vi "TAT_Com_PLC.vi"() -> ()   [LabVIEW 2017]
uses:
  NIVISION/Kapse And Sons/CKD POKAYOKE TRACIBILITY/Controls/PLC_Comm_State.ctl
  <vilib>/NI/Modbus Library/API/Master/Modbus Master.lvclass
  Global/PLC_to_Auto.vi
  <vilib>/NI/Modbus Library/API/Wrapper/Create TCP Master.vi
  <vilib>/NI/Modbus Library/API/Wrapper/API Main.lvlib
panel:
  out "s? t:f":T1
  out "Feeder Door Open":cluster{"Feeder Door Open":bool, "Address":u16}
  out "PLC IP Address":string
  out "error out 2":errorcluster
  out "error IO":errorcluster
  in  "stop 2":bool
  out "PLC STATUS station 2":bool
  out "error IO 2":errorcluster
  out "Latch Error Case":errorcluster
  out "I/O SCREEN":bool[](array[boolean])
  out "error out":errorcluster
  in  "PLC STATUS station 1":bool
  in  "error in":errorcluster
  in  "stop":bool
  # "STATION 1"
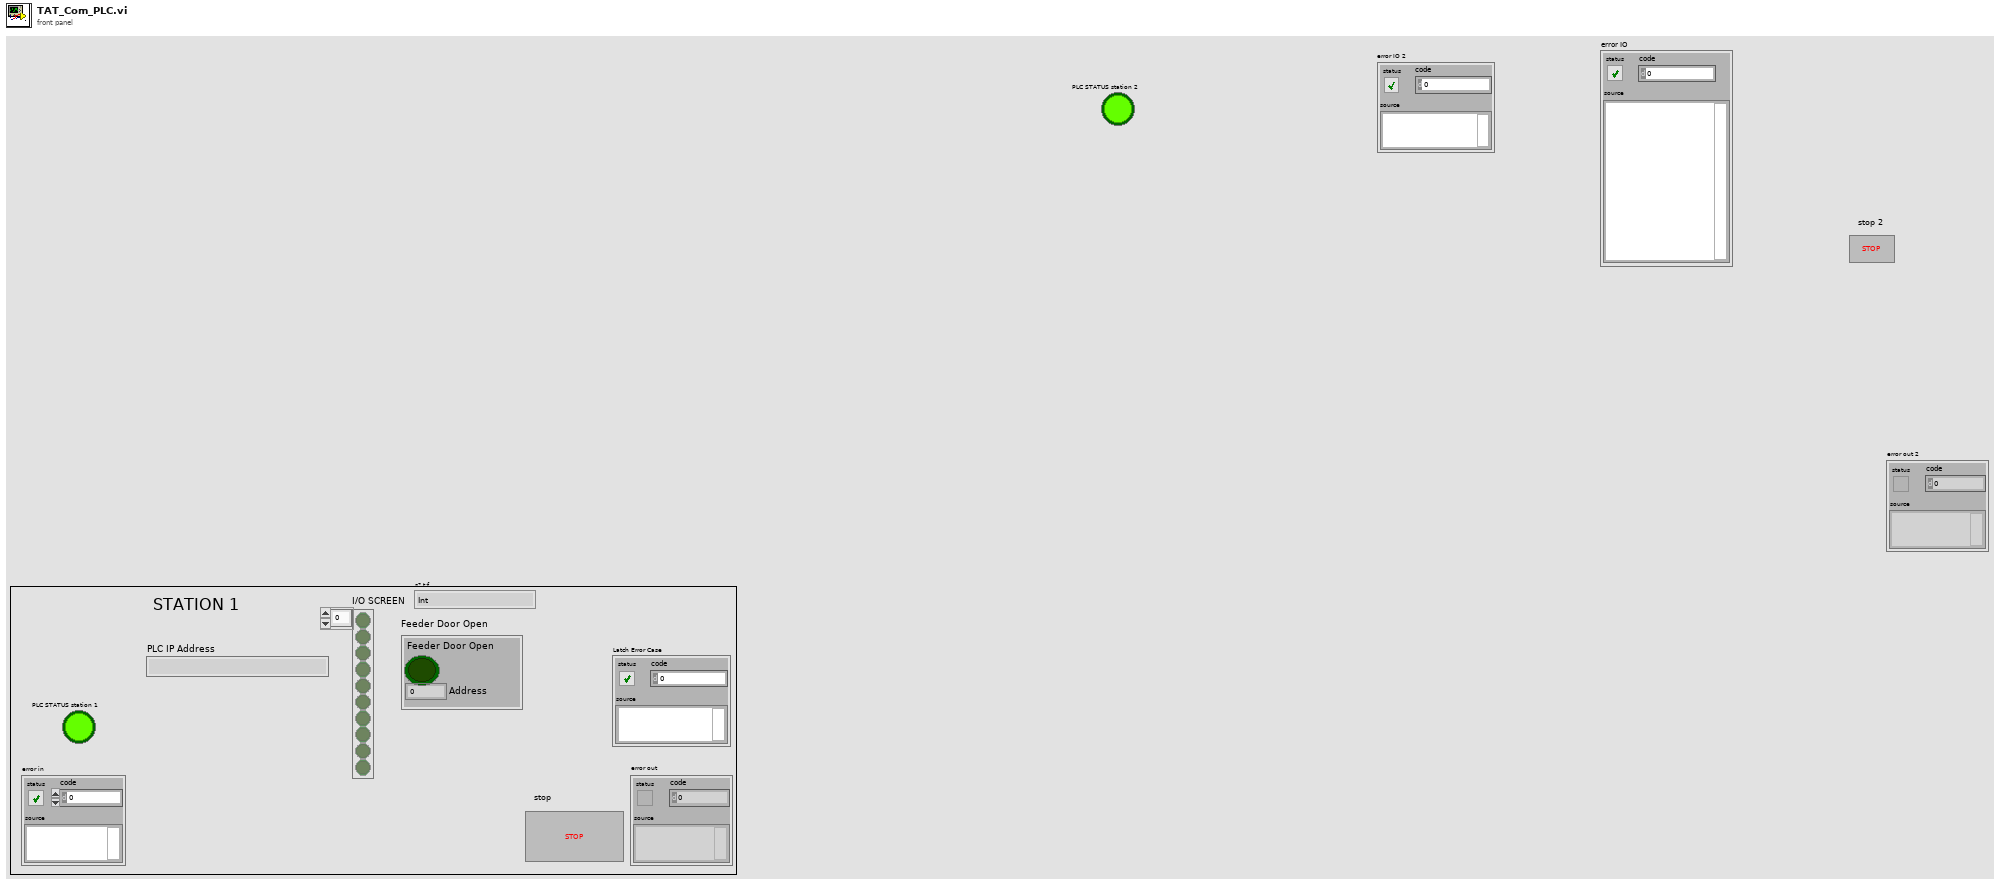
[diagram p1: front panel]
types:
  T1 = typedef "PLC_Comm_State.ctl" = enum16{"Int", "Connect", "Write", "Write2", "Write3", "Read", "Read2", "Read3", "Error", "Disconnect"}
  T2 = enum32{"invalid app kind", "Development System", "Run Time System", "Student Edition", "Embedded LabVIEW", "Evaluation", "Custom"}
  T3 = cluster{"Printer IP":string, "PLC IP Address":string, "Scanner Com":refnum<visa-resource-name>}
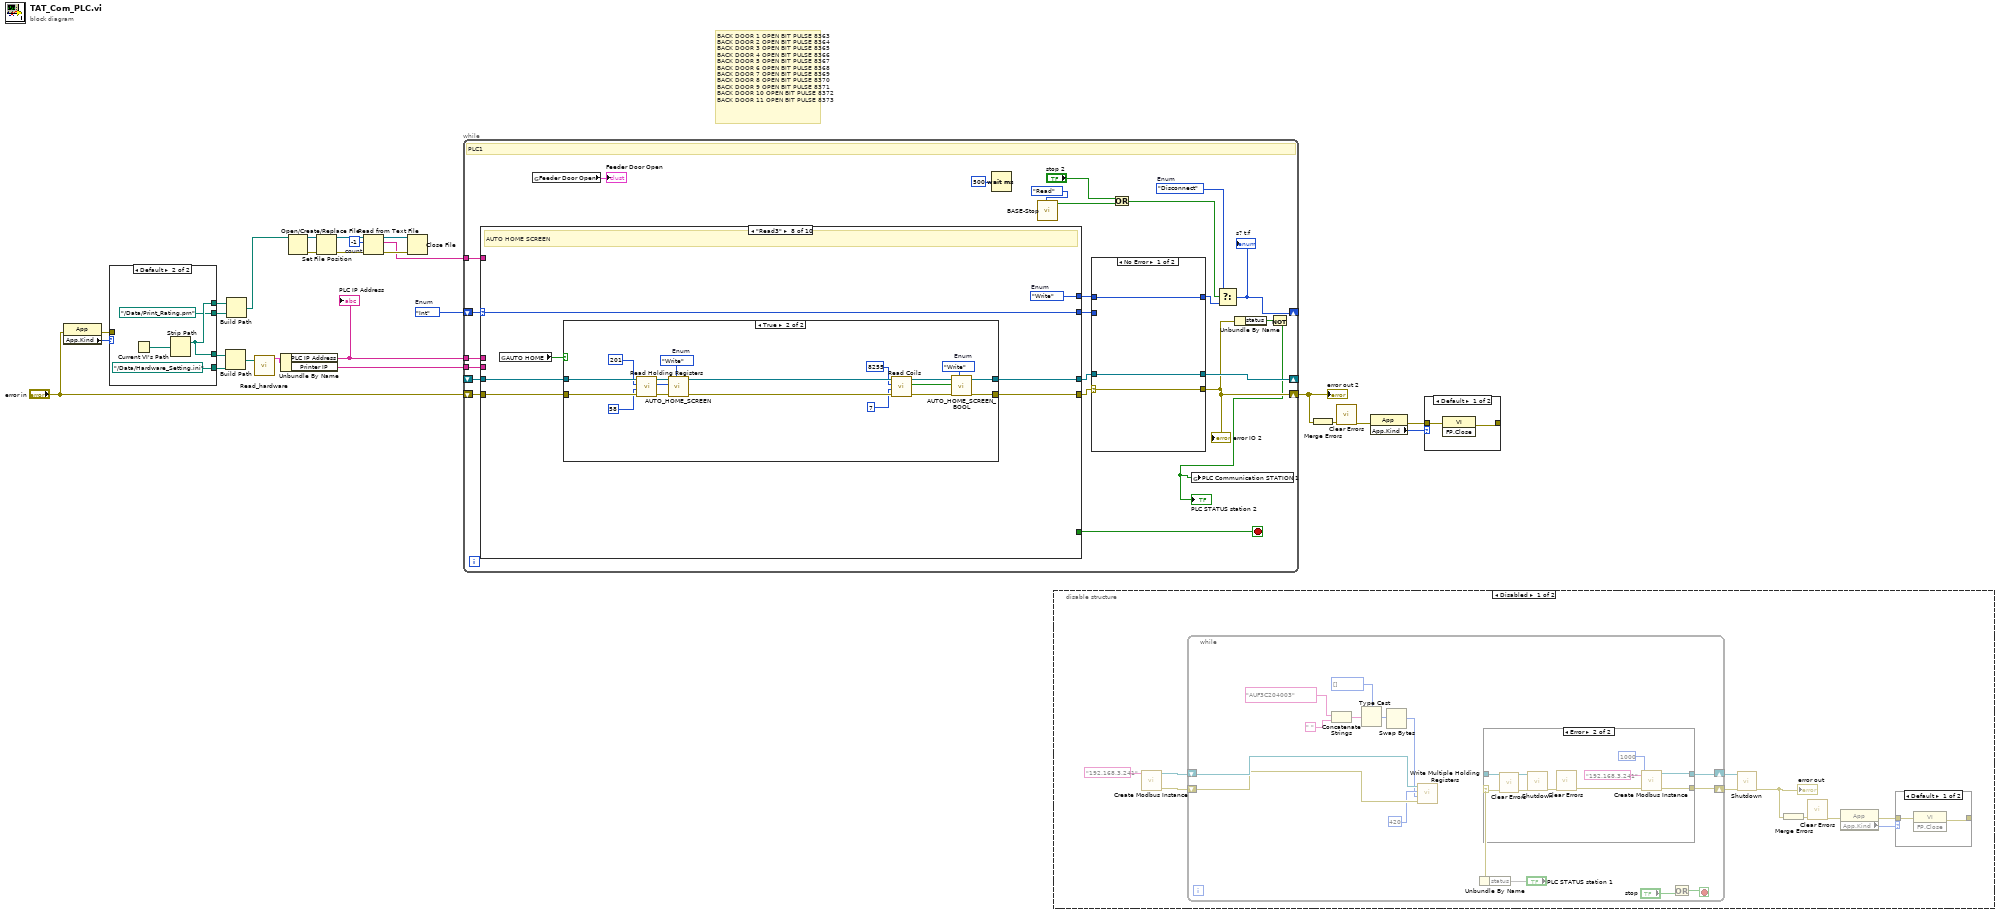
[diagram p0: block diagram]
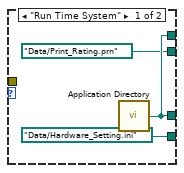
[diagram p2: hidden frame]
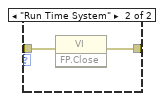
[diagram p4: hidden frame]
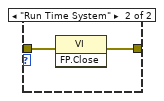
[diagram p6: hidden frame]
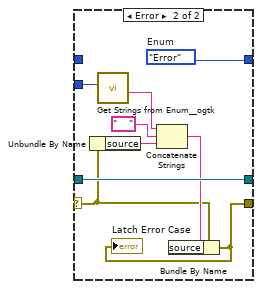
[diagram p7: hidden frame]
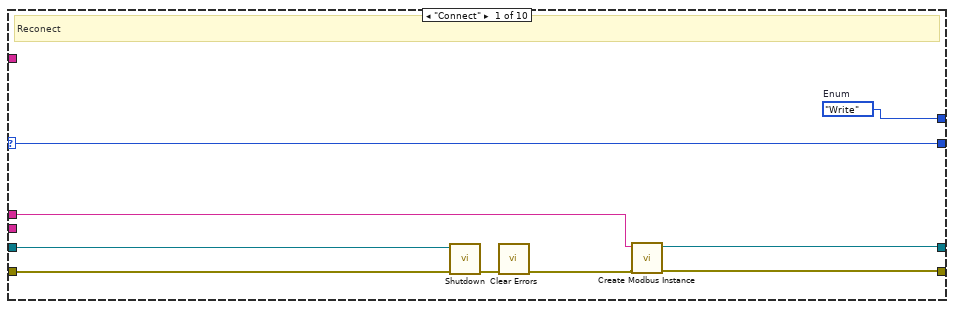
[diagram p8: hidden frame]
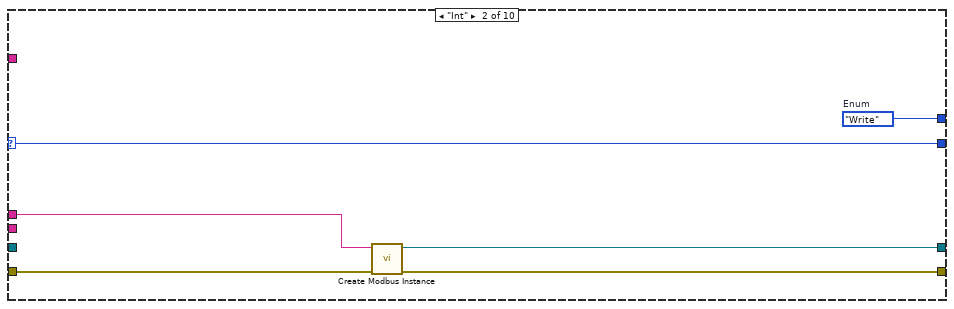
[diagram p9: hidden frame]
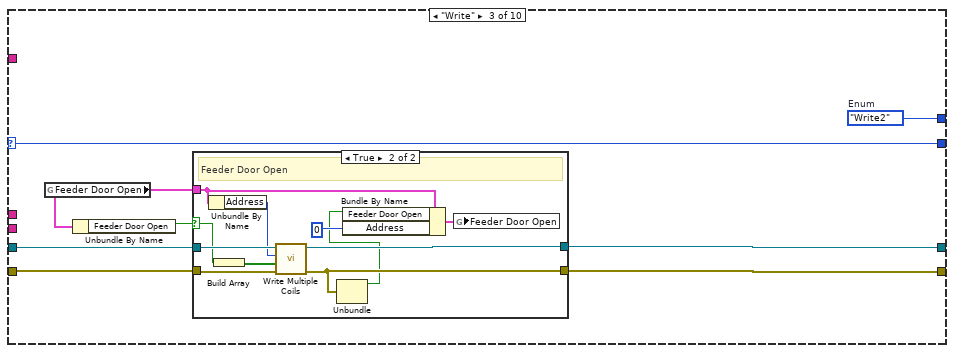
[diagram p10: hidden frame]
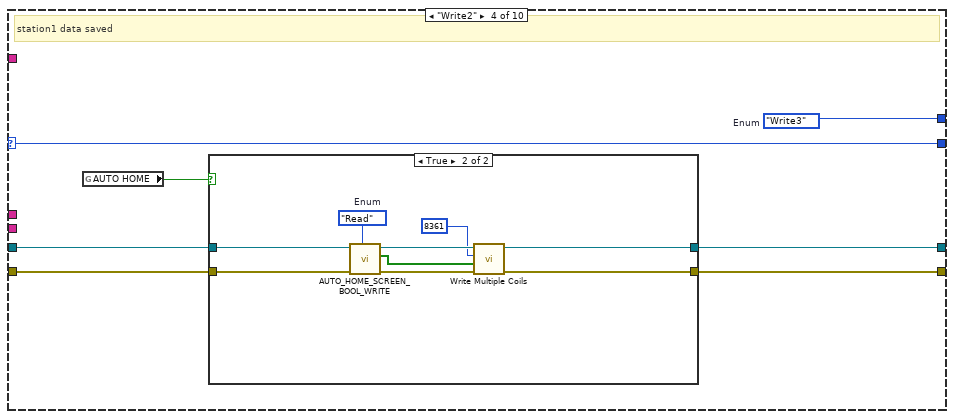
[diagram p12: hidden frame]
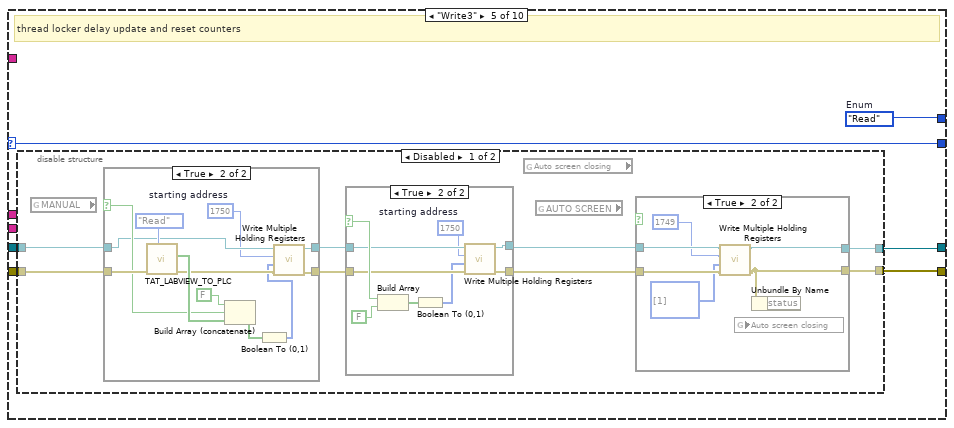
[diagram p14: hidden frame]
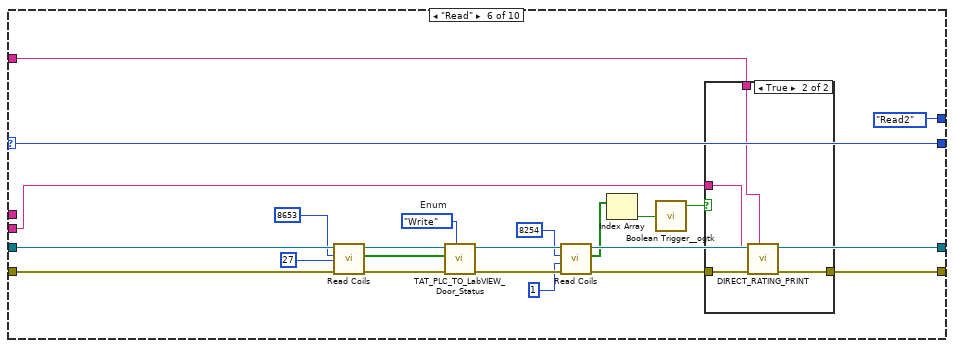
[diagram p19: hidden frame]
diagram:
  w5 = -1  # count
  w26 = PLC_Comm_State."Int"  # Enum
  # "BACK DOOR 1 OPEN BIT\tPULSE\t8363\nBACK DOOR 2 OPEN BIT\tPULSE\t8364\nBACK DOOR 3 OPEN BIT\tPULSE\t8365\nBACK DOOR 4 OPEN BIT\tPULSE\t8366\nBACK DOOR 5 OPEN BIT\tPULSE\t8367\nBACK DOOR 6 OPEN BIT\tPULSE\t8368\nBACK DOOR 7 OPEN BIT\tPULSE\t8369\nBACK DOOR 8 OPEN BIT\tPULSE\t8370\nBACK DOOR 9 OPEN BIT\tPULSE\t8371\nBACK DOOR 10 OPEN BIT\tPULSE\t8372\nBACK DOOR 11 OPEN BIT\tPULSE\t8373"
  n1 = property class="App"(error in="error in") -> (error out=w19:errorcluster, "App.Kind"=w20:T2)  [unwired: 1 in, 1 out]
  n2 = case shown="Default" w20 {
    tunnel: [w28 w31] -> w18
    tunnel: w19 -> [_ _]
    tunnel: [path "Data/Hardware_Setting.ini" ("path") path "../Data/Hardware_Setting.ini" ("path")] -> w17
    tunnel: [w28 w31] -> w4
    tunnel: [path "Data/Print_Rating.prn" ("path") path "../Data/Print_Rating.prn" ("path")] -> w3
    frame "Run Time System" {
      n3 = call <vilib>:"Application Directory.vi"() -> ("Application Directory"=w28:path)
    }
    frame Default {
      n4 = Current VI's Path() -> (path=w33:path)
      n5 = Strip Path(path=w33) -> (stripped path=w31:path)  [unwired: 1 out]
    }
  }
  n6 = Build Path(base path=w18, name or relative path=w17) -> (appended path=w16:path)
  n7 = Build Path(base path=w4, name or relative path=w3) -> (appended path=w2:path)
  n8 = call "Read_hardware.vi"("configuration file path"=w16) -> ("data"=w15:T3)  [unwired: 10 in]
  n9 = Unbundle By Name(w15) -> ("PLC IP Address"=w14:string, "Printer IP"=w12:string)
  "PLC IP Address" <- w14
  n10 = Open/Create/Replace File(file path (use dialog)=w2) -> (refnum out=w10:refnum<file>, error out=w9:errorcluster)  [unwired: 5 in, 1 out]
  n11 = Set File Position(refnum=w10, error in=w9) -> (refnum out=w8:refnum<file>, error out=w11:errorcluster)  [unwired: 2 in]
  n12 = Read from Text File(file (use dialog)=w8, count=w5, error in=w11) -> (refnum out=w7:refnum<file>, text=w1:string, error out=w6:errorcluster)  [unwired: 1 in, 1 out]
  n13 = Close File(refnum=w7, error in=w6) -> ()  [unwired: 2 out]
  n14 = while {
    shift-right: [w48] -> _
    shift-left: w26 -> [w56]
    shift-right: [w43] -> w21
    shift-left: "error in" -> [w55]
    shift-right: [w51] -> _
    shift-left: _ -> [w54]
    tunnel: w14 -> [w53]
    tunnel: w12 -> [w35]
    tunnel: w1 -> [w34]
    stop <- w49 stop-if-true
    w41 = PLC_Comm_State."Disconnect"  # Enum
    # "PLC1"
    n15 = case shown="\"Read3\"" w56 {
      selector: w56 -> [w78 w83 w92 w112 w127 w192 w202 w272 w293 w301]
      tunnel: [w75 w79 w91 w109 w123 w183 w198 w270 w294 w298] -> w57
      tunnel: [w73 w80 w90 w106 w124 w179 w199 w268 w295 w296] -> w50
      tunnel: w55 -> [w72 w84 w88 w110 w126 w188 w201 w273 w291 w303]
      tunnel: w54 -> [w70 _ w87 w107 w125 w187 w200 w269 w295 w297]
      tunnel: w53 -> [w74 w81 _ _ _ _ _ _ _ _]
      tunnel: [w77 w82 w89 w111 w128 PLC_Comm_State."Read2" ("Enum") w203 w271 w292 w300] -> w52
      tunnel: [_ _ _ _ _ _ _ _ _ TRUE] -> w49
      tunnel: [w78 w83 w92 w112 w127 w192 w202 w272 w293 w301] -> w46
      tunnel: w35 -> [_ _ _ _ _ w181 _ _ _ _]
      tunnel: w34 -> [_ _ _ _ _ w172 _ _ _ _]
      frame "Connect" {
        w77 = PLC_Comm_State."Write"  # Enum
        # "Reconect"
        n16 = call-dynamic "Shutdown.vi"("error in"=w72, "Modbus master in"=w70) -> ("error out"=w71:errorcluster)  [unwired: 9 in]
        n17 = call <vilib>:"Clear Errors.vi"("error in (no error)"=w71) -> ("error out"=w76:errorcluster)  [unwired: 5 in, 1 out]
        n18 = call-poly <vilib>:"Create Modbus Instance.vi"("error in"=w76, "address"=w74) -> ("error out"=w75:errorcluster, "TCP master instance"=w73:refnum<class "Modbus Master.lvclass">)  [unwired: 8 in]
      }
      frame "Int" {
        w82 = PLC_Comm_State."Write"  # Enum
        n19 = call-poly <vilib>:"Create Modbus Instance.vi"("error in"=w84, "address"=w81) -> ("error out"=w79:errorcluster, "TCP master instance"=w80:refnum<class "Modbus Master.lvclass">)  [unwired: 8 in]
      }
      frame "Write" {
        w89 = PLC_Comm_State."Write2"  # Enum
        n20 = global read "PLC_to_Auto.vi" "Feeder Door Open"() -> (w85:cluster{"Feeder Door Open":bool, "Address":u16})
        n21 = Unbundle By Name(w85) -> ("Feeder Door Open"=w86:bool)
        n22 = case shown="True" w86 {
          selector: w86 -> [_ w101]
          tunnel: [w93 w96] -> w91
          tunnel: w88 -> [w93 w105]
          tunnel: w87 -> [w94 w104]
          tunnel: [w94 w103] -> w90
          tunnel: w85 -> [_ w98]
          frame False {
          }
          frame True {
            # "Feeder Door Open"
            n23 = Unbundle By Name(w98) -> ("Address"=w102:u16)
            n24 = Build Array(w101) -> (w100:bool[])
            n25 = call-dynamic "Write Multiple Coils.vi"("error in"=w105, "coils to write"=w100, "starting address"=w102, "Modbus master in"=w104) -> ("error out"=w96:errorcluster, "Modbus master out"=w103:refnum<class "Modbus Master.lvclass">)  [unwired: 6 in]
            n26 = Unbundle(w96) -> ("status"=w95:bool)  [unwired: 2 out]
            n27 = Bundle By Name(cluster=w98, "Feeder Door Open"=w95, "Address"=u16 0 ("starting address")) -> (w99:cluster{"Feeder Door Open":bool, "Address":u16})
            n28 = global write "PLC_to_Auto.vi" "Feeder Door Open"(w99) -> ()
          }
        }
      }
      frame "Write2" {
        w111 = PLC_Comm_State."Write3"  # Enum
        # "station1 data saved"
        n29 = global read "PLC_to_Auto.vi" "AUTO HOME"() -> (w108:bool)
        n30 = case shown="True" w108 {
          tunnel: w110 -> [w114 w117]
          tunnel: [w114 w122] -> w109
          tunnel: w107 -> [w113 w121]
          tunnel: [w113 w120] -> w106
          frame False {
          }
          frame True {
            w118 = enum16{"Read", "Write"}."Read"  # Enum
            n31 = call "AUTO_HOME_SCREEN_BOOL_WRITE.vi"("Enum"=w118, "error in (no error)"=w117) -> ("error out"=w116:errorcluster, "Array 2"=w115:bool[])  [unwired: 8 in]
            n32 = call-dynamic "Write Multiple Coils.vi"("error in"=w116, "coils to write"=w115, "starting address"=u16 8361, "Modbus master in"=w121) -> ("error out"=w122:errorcluster, "Modbus master out"=w120:refnum<class "Modbus Master.lvclass">)  [unwired: 6 in]
          }
        }
      }
      frame "Write3" {
        w128 = PLC_Comm_State."Read"  # Enum
        # "thread locker delay update and reset counters"
        n33 = disable-structure shown="Disabled" {
          disable-tunnel: w126 -> [w136 w170]
          disable-tunnel: w125 -> [w135 w171]
          disable-tunnel: [w132 w171] -> w124
          disable-tunnel: [w131 w170] -> w123
          frame Disabled {
            n34 = global read "PLC_to_Auto.vi" "MANUAL"() -> ()  [unwired: 1 out]
            n35 = case shown="True" {
              selector: _ -> [_ w166]
              tunnel: w136 -> [w156 w168]
              tunnel: w135 -> [w157 w160]
              tunnel: [w157 w161] -> w133
              tunnel: [w156 w163] -> w134
              frame False {
              }
              frame True {
                w159 = u16 1750  # starting address
                n36 = call "TAT_LABVIEW_TO_PLC.vi"("Enum"=enum16{"Read", "Write"}."Read", "error in (no error)"=w168) -> ("error out"=w162:errorcluster, "Array 2"=w167:bool[])  [unwired: 8 in]
                n37 = Build Array (concatenate)(FALSE, w166, w167) -> (w164:bool[])
                n38 = Boolean To (0,1)(Boolean=w164) -> (0, 1=w158:i16[])
                n39 = call-dynamic "Write Multiple Holding Registers.vi"("error in"=w162, "registers to write"=w158, "starting address"=w159, "Modbus master in"=w160) -> ("error out"=w163:errorcluster, "Modbus master out"=w161:refnum<class "Modbus Master.lvclass">)  [unwired: 6 in]
              }
            }
            n40 = case shown="True" {
              selector: _ -> [_ w155]
              tunnel: w134 -> [w146 w153]
              tunnel: [w146 w152] -> w130
              tunnel: w133 -> [w145 w151]
              tunnel: [w145 w150] -> w129
              frame False {
              }
              frame True {
                w147 = u16 1750  # starting address
                n41 = Build Array(w155, FALSE) -> (w148:bool[])
                n42 = Boolean To (0,1)(Boolean=w148) -> (0, 1=w149:i16[])
                n43 = call-dynamic "Write Multiple Holding Registers.vi"("error in"=w153, "registers to write"=w149, "starting address"=w147, "Modbus master in"=w151) -> ("error out"=w152:errorcluster, "Modbus master out"=w150:refnum<class "Modbus Master.lvclass">)  [unwired: 6 in]
              }
            }
            n44 = global read "PLC_to_Auto.vi" "Auto screen closing"() -> ()  [unwired: 1 out]
            n45 = global read "PLC_to_Auto.vi" "AUTO SCREEN"() -> ()  [unwired: 1 out]
            n46 = case shown="True" {
              selector: _ -> [_ _]
              tunnel: [w137 w142] -> w132
              tunnel: [w138 w143] -> w131
              tunnel: w129 -> [w137 w141]
              tunnel: w130 -> [w138 w144]
              frame False {
              }
              frame True {
                n47 = call-dynamic "Write Multiple Holding Registers.vi"("error in"=w144, "registers to write"=u16[] [1], "starting address"=u16 1749, "Modbus master in"=w141) -> ("error out"=w143:errorcluster, "Modbus master out"=w142:refnum<class "Modbus Master.lvclass">)  [unwired: 6 in]
                n48 = global read "PLC_to_Auto.vi" "Auto screen closing"() -> ()  [unwired: 1 in]
                n49 = Unbundle By Name(w143) -> ()  [unwired: 1 out]
              }
            }
          }
          frame Enabled {
          }
        }
      }
      frame "Read" {
        w190 = enum16{"Read", "Write"}."Write"  # Enum
        n50 = call-dynamic "Read Coils.vi"("error in"=w188, "number of inputs"=u16 27, "starting address"=u16 8653, "Modbus master in"=w187) -> ("error out"=w189:errorcluster, "coils"=w184:bool[], "Modbus master out"=w180:refnum<class "Modbus Master.lvclass">)  [unwired: 5 in]
        n51 = call "TAT_PLC_TO_LabVIEW_Door_Status.vi"("Enum"=w190, "error in (no error)"=w189, "Array"=w184) -> ("error out"=w178:errorcluster)  [unwired: 7 in, 1 out]
        n52 = call-dynamic "Read Coils.vi"("error in"=w178, "number of inputs"=u16 1, "starting address"=u16 8254, "Modbus master in"=w180) -> ("error out"=w177:errorcluster, "coils"=w174:bool[], "Modbus master out"=w179:refnum<class "Modbus Master.lvclass">)  [unwired: 5 in]
        n53 = Index Array(array=w174) -> (element=w173:bool)  [unwired: 1 in]
        n54 = call <userlib>:"Boolean Trigger__ogtk.vi"("Boolean Input"=w173) -> ("Rising Edge"=w182:bool)  [unwired: 1 in, 1 out]
        n55 = case shown="True" w182 {
          tunnel: w177 -> [w193 w197]
          tunnel: [w193 w196] -> w183
          tunnel: w181 -> [_ w195]
          tunnel: w172 -> [_ w194]
          frame False {
          }
          frame True {
            n56 = call "DIRECT_RATING_PRINT.vi"("PRN Data"=w194, "error in"=w197, "Printer IP"=w195) -> ("error out"=w196:errorcluster)  [unwired: 8 in]
          }
        }
      }
      frame "Read2" {
        w203 = PLC_Comm_State."Read3"  # Enum
        # "I/O SCREEN INDICATORS"
        n57 = disable-structure shown="Enabled" {
          disable-tunnel: w201 -> [w208 w223]
          disable-tunnel: w200 -> [w207 w220]
          disable-tunnel: [w206 w221] -> w199
          disable-tunnel: [w205 w222] -> w198
          frame Disabled {
            # "D1551"
            n58 = call "Elapsed Time"() -> ("Time has Elapsed"=w204:bool)  [unwired: 12 in, 7 out]
            n59 = case shown="True" w204 {
              tunnel: w208 -> [w209 w217]
              tunnel: w207 -> [w210 w216]
              tunnel: [w210 w215] -> w206
              tunnel: [w209 w211] -> w205
              frame False {
              }
              frame True {
                w214 = enum16{"Read", "Write"}."Write"  # Enum
                w219 = u16 5  # number of inputs
                n60 = call-dynamic "Read Coils.vi"("error in"=w217, "number of inputs"=w219, "starting address"=u16 3000, "Modbus master in"=w216) -> ("error out"=w212:errorcluster, "coils"=w213:bool[], "Modbus master out"=w215:refnum<class "Modbus Master.lvclass">)  [unwired: 5 in]
                n61 = call "TAT_PLC_Data_read_Indictors.vi"("Enum"=w214, "error in (no error)"=w212, "Array"=w213) -> ("error out"=w211:errorcluster)  [unwired: 7 in, 1 out]
              }
            }
          }
          frame Enabled {
            n62 = global read "PLC_to_Auto.vi" "I/O MANUAL ON"() -> (w228:bool)
            n63 = case shown="True" w228 {
              tunnel: w223 -> [w229 w238]
              tunnel: [w229 w233] -> w224
              tunnel: [w230 w232] -> w225
              tunnel: w220 -> [w230 w241]
              frame False {
                # "Manual screen OFF"
              }
              frame True {
                # "Manual screen ON"
                n64 = call "TAT_LABVIEW_TO_PLC.vi"("Enum"=enum16{"Read", "Write"}."Read", "error in (no error)"=w238) -> ("error out"=w237:errorcluster, "Array 2"=w236:bool[])  [unwired: 8 in]
                n65 = Or Array Elements(Boolean array=w236) -> (logical OR=w235:bool)
                n66 = call-dynamic "Write Multiple Coils.vi"("error in"=w237, "coils to write"=w236, "starting address"=u16 8393, "Modbus master in"=w241) -> ("error out"=w234:errorcluster, "Modbus master out"=w231:refnum<class "Modbus Master.lvclass">)  [unwired: 6 in]
                n67 = case shown="True" w235 {
                  tunnel: w234 -> [w242 w248]
                  tunnel: [w242 w247] -> w233
                  tunnel: [w243 w246] -> w232
                  tunnel: w231 -> [w243 w246]
                  frame False {
                  }
                  frame True {
                    n68 = call "TAT_LABVIEW_TO_PLC.vi"("Enum"=enum16{"Read", "Write"}."Write", "error in (no error)"=w248, "Array"=bool[] [FALSE, FALSE, FALSE, FALSE, FALSE, FALSE, FALSE, FALSE, FALSE, FALSE, FALSE, FALSE, FALSE, FALSE, FALSE, FALSE, FALSE, FALSE, FALSE, FALSE, FALSE, FALSE, FALSE, FALSE, FALSE, FALSE, FALSE, FALSE, FALSE, FALSE, FALSE, FALSE, FALSE, FALSE, FALSE, FALSE, FALSE, FALSE, FALSE, FALSE, FALSE, FALSE, FALSE, FALSE, FALSE]) -> ("error out"=w247:errorcluster)  [unwired: 7 in, 1 out]
                  }
                }
              }
            }
            n69 = global read "PLC_to_Auto.vi" "I/O SCREEN ON"() -> (w226:bool)
            n70 = Or(x=w228, y=w226) -> (x .or. y?=w227:bool)
            n71 = case shown="True" w227 {
              tunnel: [w249 w254] -> w222
              tunnel: [w250 w259] -> w221
              tunnel: w224 -> [w249 w257]
              tunnel: w225 -> [w250 w256]
              frame False {
                # "I/O SCREEN Off-"
              }
              frame True {
                w258 = u16[] [8192, 8202, 8212, 8222, 8232, 8292, 8302, 8312, 8322, 8332]  # starting address 3
                w255 = enum16{"Read", "Write"}."Write"  # Enum
                # "I/O SCREEN ON-"
                n72 = for {
                  tunnel: u16 8 ("number of inputs") -> [w263]
                  tunnel: w258 -> [w262] mode=indexing
                  tunnel: w257 -> [w266]
                  tunnel: [w261] -> w253
                  tunnel: w256 -> [w265]
                  tunnel: [w264] -> w259
                  tunnel: [w260] -> w252 mode=concatenating
                  n73 = call-dynamic "Read Coils.vi"("error in"=w266, "number of inputs"=w263, "starting address"=w262, "Modbus master in"=w265) -> ("error out"=w261:errorcluster, "coils"=w260:bool[], "Modbus master out"=w264:refnum<class "Modbus Master.lvclass">)  [unwired: 5 in]
                }
                "I/O SCREEN" <- w252
                n74 = call "TAT_PLC_Data_read_BOLLEAN_I_O_SCREEN.vi"("Enum"=w255, "error in (no error)"=w253, "Array"=w252) -> ("error out"=w254:errorcluster)  [unwired: 7 in, 1 out]
              }
            }
          }
        }
      }
      frame "Read3" {
        w271 = PLC_Comm_State."Write"  # Enum
        # "AUTO HOME SCREEN"
        n75 = global read "PLC_to_Auto.vi" "AUTO HOME"() -> (w267:bool)
        n76 = case shown="True" w267 {
          tunnel: w273 -> [w274 w290]
          tunnel: [w274 w281] -> w270
          tunnel: w269 -> [w275 w289]
          tunnel: [w275 w279] -> w268
          frame False {
          }
          frame True {
            w283 = enum16{"Read", "Write"}."Write"  # Enum
            w285 = enum16{"Read", "Write"}."Write"  # Enum
            n77 = call-dynamic "Read Holding Registers.vi"("error in"=w290, "number of inputs"=u16 58, "starting address"=u16 201, "Modbus master in"=w289) -> ("error out"=w286:errorcluster, "register values"=w284:u16[], "Modbus master out"=w280:refnum<class "Modbus Master.lvclass">)  [unwired: 5 in]
            n78 = call "AUTO_HOME_SCREEN.vi"("Enum"=w285, "error in (no error)"=w286, "Array"=w284) -> ("error out"=w282:errorcluster)  [unwired: 7 in, 1 out]
            n79 = call-dynamic "Read Coils.vi"("error in"=w282, "number of inputs"=u16 7, "starting address"=u16 8255, "Modbus master in"=w280) -> ("error out"=w281:errorcluster, "coils"=w276:bool[], "Modbus master out"=w279:refnum<class "Modbus Master.lvclass">)  [unwired: 5 in]
            n80 = call "AUTO_HOME_SCREEN_BOOL.vi"("Enum"=w283, "Array"=w276) -> ()  [unwired: 8 in, 2 out]
          }
        }
      }
      frame "Error" {
        w292 = PLC_Comm_State."Connect"  # Enum
        n81 = call <vilib>:"Clear Errors.vi"("error in (no error)"=w291) -> ("error out"=w294:errorcluster)  [unwired: 5 in, 1 out]
        "error IO" <- w291
      }
      frame "Disconnect" {
        w296 = refnum<class "Modbus Master.lvclass"> refnum  # Modbus master out
        w300 = PLC_Comm_State."Disconnect"  # Enum
        n82 = call <vilib>:"Clear Errors.vi"("error in (no error)"=w303) -> ("error out"=w299:errorcluster)  [unwired: 5 in, 1 out]
        n83 = call-dynamic "Shutdown.vi"("error in"=w299, "Modbus master in"=w297) -> ("error out"=w298:errorcluster)  [unwired: 9 in]
      }
    }
    n84 = global read "PLC_to_Auto.vi" "Feeder Door Open"() -> (→"Feeder Door Open":cluster{"Feeder Door Open":bool, "Address":u16})
    n85 = Wait (ms)(milliseconds to wait=u32 500) -> ()  [unwired: 1 out]
    n86 = call "BASE-Stop.vi"("Enum"=enum16{"Read", "Write"}."Read") -> ("Stop"=w39:bool)  [unwired: 10 in]
    n87 = case shown="No Error" w57 {
      selector: w57 -> [w60 w63]
      tunnel: [w60 w61] -> w43
      tunnel: [w59 w62] -> w47
      tunnel: w52 -> [w59 _]
      tunnel: [w58 w69] -> w51
      tunnel: w50 -> [w58 w69]
      tunnel: w46 -> [_ w67]
      frame No Error {
      }
      frame Error {
        w62 = PLC_Comm_State."Error"  # Enum
        n88 = Unbundle By Name(w63) -> ("source"=w68:string)
        n89 = call <userlib>:"Get Strings from Enum__ogtk.vi"("Enum"=w67) -> ("String Value"=w66:string)  [unwired: 7 in, 3 out]
        n90 = Concatenate Strings(w66, "    " ("string"), w68) -> (w64:string)
        n91 = Bundle By Name(cluster=w63, "source"=w64) -> (w61:errorcluster)
        "Latch Error Case" <- w61
      }
    }
    "error IO 2" <- w43
    n92 = Or(x="stop 2", y=w39) -> (x .or. y?=w45:bool)
    n93 = Select(t=w41, s=w45, f=w47) -> (s? t:f=w48:T1)
    "s? t:f" <- w48
    n94 = Unbundle By Name(w43) -> ("status"=w44:bool)
    n95 = Not(x=w44) -> (.not. x?=w38:bool)
    "PLC STATUS station 2" <- w38
    n96 = global write "PLC_to_Auto.vi" "PLC Communication STATION 1"(w38) -> ()
  }
  "error out 2" <- w21
  n97 = disable-structure shown="Disabled" {
    frame Disabled {
      n98 = call-poly <vilib>:"Create Modbus Instance.vi"("address"="192.168.3.241") -> ("error out"=w308:errorcluster, "TCP master instance"=w307:refnum<class "Modbus Master.lvclass">)  [unwired: 9 in]
      n99 = while {
        shift-right: [w329] -> w312
        shift-left: w307 -> [w323]
        shift-right: [w328] -> w311
        shift-left: w308 -> [w321]
        stop <- w330 stop-if-true
        n100 = Concatenate Strings("AUF3C204003", " ") -> (w314:string)
        n101 = Type Cast(type=u16[] [] ("Register"), x=w314) -> (*(type *) &x=w317:u16[])
        n102 = Swap Bytes(anything=w317) -> (byte swapped=w316:u16[])
        n103 = call-dynamic "Write Multiple Holding Registers.vi"("error in"=w321, "registers to write"=w316, "starting address"=u16 420, "Modbus master in"=w323) -> ("error out"=w320:errorcluster, "Modbus master out"=w322:refnum<class "Modbus Master.lvclass">)  [unwired: 6 in]
        n104 = case shown="Error" w325 {
          selector: [w332 w342] -> w325
          tunnel: [w333 w340] -> w327
          tunnel: [w333 w336] -> w329
          tunnel: [w332 w335] -> w328
          frame No Error {
          }
          frame Error {
            n105 = call <vilib>:"Clear Errors.vi"("error in (no error)"=w342) -> ("error out"=w341:errorcluster)  [unwired: 5 in, 1 out]
            n106 = call-dynamic "Shutdown.vi"("error in"=w341, "Modbus master in"=w340) -> ("error out"=w339:errorcluster)  [unwired: 9 in]
            n107 = call <vilib>:"Clear Errors.vi"("error in (no error)"=w339) -> ("error out"=w337:errorcluster)  [unwired: 5 in, 1 out]
            n108 = call-poly <vilib>:"Create Modbus Instance.vi"("error in"=w337, "connect timeout ms"=1000, "address"="192.168.3.241") -> ("error out"=w335:errorcluster, "TCP master instance"=w336:refnum<class "Modbus Master.lvclass">)  [unwired: 7 in]
          }
        }
        n109 = Unbundle By Name(w325) -> ("status"=→"PLC STATUS station 1")
        n110 = Or(y="stop") -> (x .or. y?=w330:bool)  [unwired: 1 in]
      }
      n111 = call-dynamic "Shutdown.vi"("error in"=w311, "Modbus master in"=w312) -> ("error out"=w305:errorcluster)  [unwired: 9 in]
      "error out" <- w305
      n112 = Merge Errors(w305) -> (w304:errorcluster)
      n113 = call <vilib>:"Clear Errors.vi"("error in (no error)"=w304) -> ("error out"=w306:errorcluster)  [unwired: 5 in, 1 out]
      n114 = property class="App"(error in=w306) -> (error out=w309:errorcluster, "App.Kind"=w310:T2)  [unwired: 1 in, 1 out]
      n115 = case shown="Default" w310 {
        tunnel: w309 -> [w344 w346]
        tunnel: [w343 w345] -> _
        frame Default {
          n116 = invoke class="VI" method="FP.Close"(error in=w344) -> (error out=w343:errorcluster)  [unwired: 2 in, 2 out]
        }
        frame "Run Time System" {
          n117 = invoke class="VI" method="FP.Close"(error in=w346) -> (error out=w345:errorcluster)  [unwired: 2 in, 2 out]
        }
      }
    }
    frame Enabled {
    }
  }
  n118 = Merge Errors(w21) -> (w25:errorcluster)
  n119 = call <vilib>:"Clear Errors.vi"("error in (no error)"=w25) -> ("error out"=w24:errorcluster)  [unwired: 5 in, 1 out]
  n120 = property class="App"(error in=w24) -> (error out=w23:errorcluster, "App.Kind"=w22:T2)  [unwired: 1 in, 1 out]
  n121 = case shown="Default" w22 {
    tunnel: w23 -> [w348 w350]
    tunnel: [w347 w349] -> _
    frame Default {
      n122 = invoke class="VI" method="FP.Close"(error in=w348) -> (error out=w347:errorcluster)  [unwired: 2 in, 2 out]
    }
    frame "Run Time System" {
      n123 = invoke class="VI" method="FP.Close"(error in=w350) -> (error out=w349:errorcluster)  [unwired: 2 in, 2 out]
    }
  }
